vi "Sequence.CreateStepLoop.vi"(7 "Iteration":string, 8 "error in (no error)":errorcluster, 10 "Duration":dbl, 11 "Elements":T1[](array[typedef])) -> (0 "error out":errorcluster, 3 "Tasks":refnum<k24>[](array[refnum]))   [LabVIEW 2015, in "Single Station Execution.lvlib"]
uses:
  Single Station Execution.lvlib
  NationalInstruments.VeriStand.RealTimeSequenceDefinitionApi
  Main.Constants.vi
  Types/Step.Types.ctl
  Types/Channel.Properties.ctl
  Types/Compiled.StepElementProperties.ctl
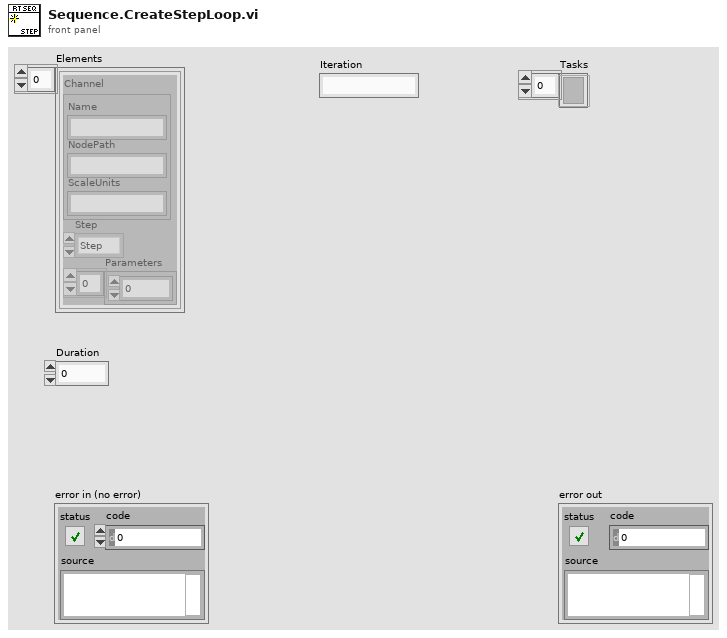
[diagram p1: front panel]
types:
  T1 = typedef "Single Station Execution.lvlib/Compiled.StepElementProperties.ctl" = cluster{"Channel":T2, "Step":T3, "Parameters":dbl[]}
  T2 = typedef "Single Station Execution.lvlib/Channel.Properties.ctl" = cluster{"Name":string, "NodePath":string, "ScaleUnits":string}
  T3 = typedef "Single Station Execution.lvlib/Step.Types.ctl" = enum8{"Step", "iStep", "Ramp", "Unchanged", "Unknown", "Sine", "LogSine", "LinearSine", "ForcedRamp", "Waveform"}
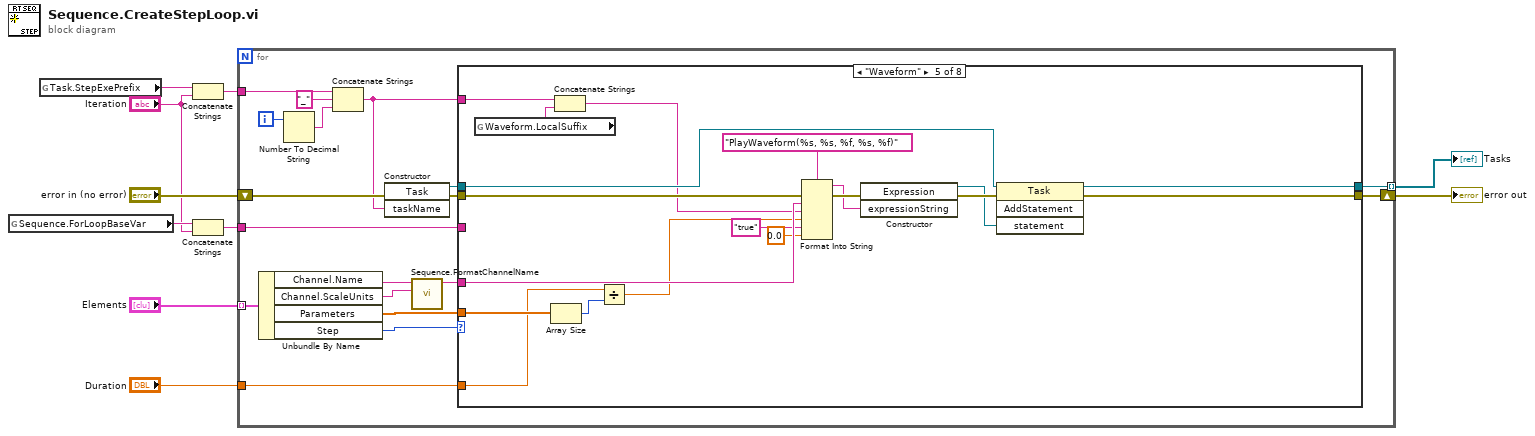
[diagram p0: block diagram]
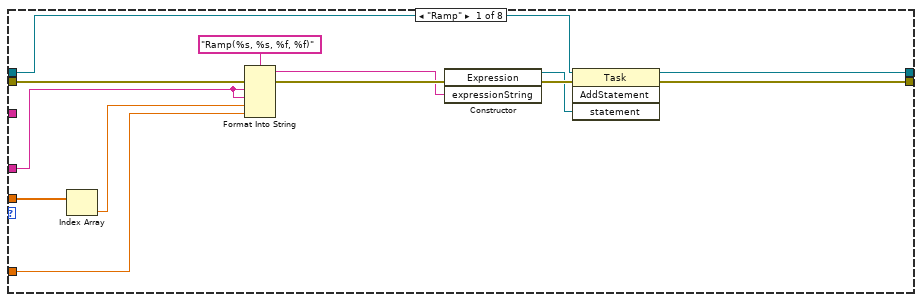
[diagram p2: hidden frame]
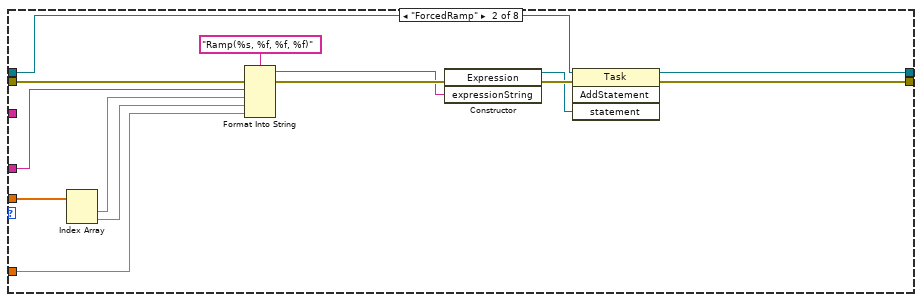
[diagram p3: hidden frame]
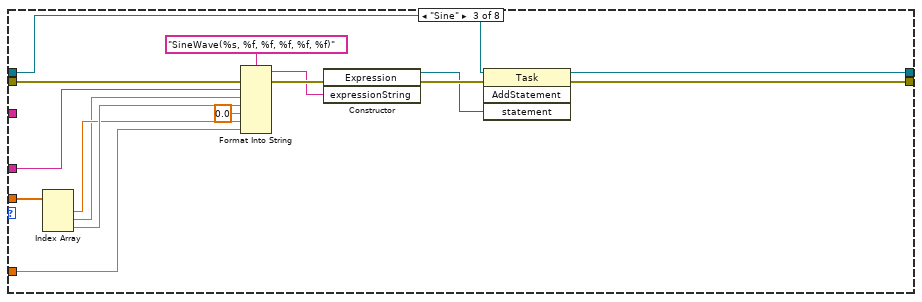
[diagram p4: hidden frame]
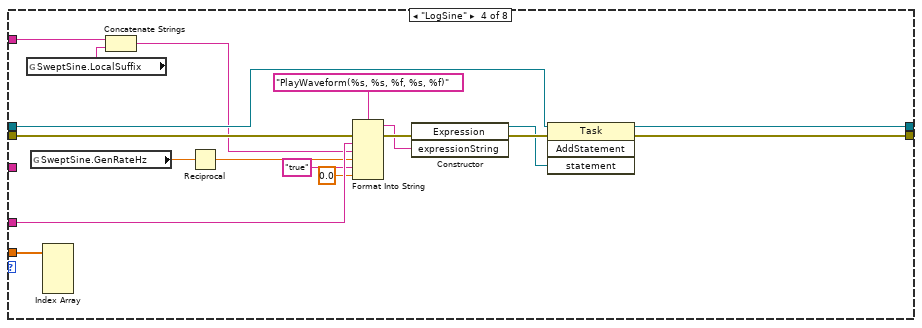
[diagram p5: hidden frame]
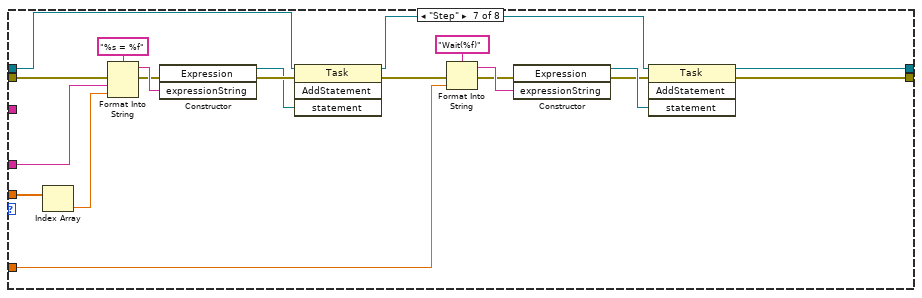
[diagram p7: hidden frame]
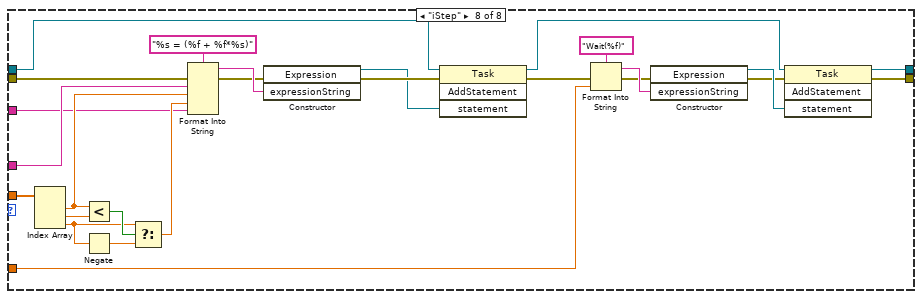
[diagram p8: hidden frame]
diagram:
  n1 = global read "Main.Constants.vi" "Sequence.ForLoopBaseVar"() -> (w3:string)
  n2 = global read "Main.Constants.vi" "Task.StepExePrefix"() -> (w5:string)
  n3 = Concatenate Strings(w5, "Iteration") -> (w4:string)
  n4 = Concatenate Strings(w3, "Iteration") -> (w1:string)
  n5 = for {
    tunnel: "Elements" -> [w24] mode=indexing
    shift-right: [w15] -> w9
    shift-left: "error in (no error)" -> [w23]
    tunnel: w4 -> [w27]
    tunnel: [w13] -> w10 mode=indexing
    tunnel: "Duration" -> [w19]
    tunnel: w1 -> [w12]
    i -> [w28]
    n6 = Unbundle By Name(w24) -> ("Channel.Name"=w22:string, "Channel.ScaleUnits"=w21:string, "Parameters"=w18:dbl[], "Step"=w17:T3)
    n7 = Number To Decimal String(number=w28) -> (decimal integer string=w25:string)  [unwired: 1 in]
    n8 = Concatenate Strings(w27, "_" ("string"), w25) -> (w11:string)
    n9 = constructor class="Task"(error in=w23, "taskName"=w11) -> (reference out=w14:refnum<k24>, error out=w16:errorcluster)  [unwired: 2 in, 2 out]
    n10 = call "Sequence.FormatChannelName.vi"("ScaleUnits"=w21, "Name"=w22) -> ("ChannelName"=w20:string)  [unwired: 9 in]
    n11 = case shown="\"Waveform\"" w17 {
      tunnel: w20 -> [w41 w55 w70 w88 w107 _ w129 w155]
      tunnel: w18 -> [w30 w43 w69 w87 w92 _ w128 w154]
      tunnel: w19 -> [w39 w52 w58 _ w90 _ w119 w146]
      tunnel: [w33 w46 w63 w81 w101 w109 w113 w140] -> w15
      tunnel: w16 -> [w38 w51 w68 w86 w106 w109 w126 w153]
      tunnel: w14 -> [w35 w48 w65 w83 w103 w110 w118 w145]
      tunnel: [w32 w45 w62 w80 w100 w110 w111 w138] -> w13
      tunnel: w12 -> [_ _ _ _ _ _ _ w131]
      tunnel: w11 -> [_ _ _ w75 w96 _ _ _]
      frame "Ramp" {
        n12 = Index Array(array=w30) -> (element=w40:dbl)  [unwired: 1 in]
        n13 = Format Into String(format string="Ramp(%s, %s, %f, %f)" ("expressionString"), error in=w38, w41, w41, w40, w39) -> (resulting string=w31:string, error out=w34:errorcluster)  [unwired: 1 in]
        n14 = constructor class="Expression"(error in=w34, "expressionString"=w31) -> (reference out=w36:refnum<k24>, error out=w37:errorcluster)  [unwired: 2 in, 2 out]
        n15 = invoke class="Task" method="AddStatement"(reference=w35, error in=w37, "statement"=w36) -> (reference out=w32:refnum<k24>, error out=w33:errorcluster)  [unwired: 1 in, 2 out]
      }
      frame "ForcedRamp" {
        n16 = Index Array(array=w43) -> (element #1=w54:dbl, element #2=w53:dbl)  [unwired: 2 in]
        n17 = Format Into String(format string="Ramp(%s, %f, %f, %f)" ("expressionString"), error in=w51, w55, w54, w53, w52) -> (resulting string=w44:string, error out=w47:errorcluster)  [unwired: 1 in]
        n18 = constructor class="Expression"(error in=w47, "expressionString"=w44) -> (reference out=w49:refnum<k24>, error out=w50:errorcluster)  [unwired: 2 in, 2 out]
        n19 = invoke class="Task" method="AddStatement"(reference=w48, error in=w50, "statement"=w49) -> (reference out=w45:refnum<k24>, error out=w46:errorcluster)  [unwired: 1 in, 2 out]
      }
      frame "Sine" {
        n20 = Index Array(array=w69) -> (element #1=w57:dbl, element #2=w56:dbl, element #3=w60:dbl)  [unwired: 3 in]
        n21 = Format Into String(format string="SineWave(%s, %f, %f, %f, %f, %f)" ("expressionString"), error in=w68, w70, w56, w60, 0.0 ("input 4"), w57, w58) -> (resulting string=w61:string, error out=w64:errorcluster)  [unwired: 1 in]
        n22 = constructor class="Expression"(error in=w64, "expressionString"=w61) -> (reference out=w66:refnum<k24>, error out=w67:errorcluster)  [unwired: 2 in, 2 out]
        n23 = invoke class="Task" method="AddStatement"(reference=w65, error in=w67, "statement"=w66) -> (reference out=w62:refnum<k24>, error out=w63:errorcluster)  [unwired: 1 in, 2 out]
      }
      frame "LogSine" {
        n24 = global read "Main.Constants.vi" "SweptSine.LocalSuffix"() -> (w73:string)
        n25 = global read "Main.Constants.vi" "SweptSine.GenRateHz"() -> (w72:dbl)
        n26 = Index Array(array=w87) -> ()  [unwired: 4 in, 4 out]
        n27 = Concatenate Strings(w75, w73) -> (w74:string)
        n28 = Reciprocal(x=w72) -> (1/x=w76:dbl)
        n29 = Format Into String(format string="PlayWaveform(%s, %s, %f, %s, %f)" ("expressionString"), error in=w86, w88, w74, w76, "true" ("input 4"), 0.0 ("input 4")) -> (resulting string=w79:string, error out=w82:errorcluster)  [unwired: 1 in]
        n30 = constructor class="Expression"(error in=w82, "expressionString"=w79) -> (reference out=w84:refnum<k24>, error out=w85:errorcluster)  [unwired: 2 in, 2 out]
        n31 = invoke class="Task" method="AddStatement"(reference=w83, error in=w85, "statement"=w84) -> (reference out=w80:refnum<k24>, error out=w81:errorcluster)  [unwired: 1 in, 2 out]
      }
      frame "Waveform" {
        n32 = global read "Main.Constants.vi" "Waveform.LocalSuffix"() -> (w94:string)
        n33 = Array Size(array=w92) -> (size(s)=w93:i32)
        n34 = Concatenate Strings(w96, w94) -> (w95:string)
        n35 = Divide(x=w90, y=w93) -> (x/y=w91:dbl)
        n36 = Format Into String(format string="PlayWaveform(%s, %s, %f, %s, %f)" ("expressionString"), error in=w106, w107, w95, w91, "true" ("input 4"), 0.0 ("input 4")) -> (resulting string=w99:string, error out=w102:errorcluster)  [unwired: 1 in]
        n37 = constructor class="Expression"(error in=w102, "expressionString"=w99) -> (reference out=w104:refnum<k24>, error out=w105:errorcluster)  [unwired: 2 in, 2 out]
        n38 = invoke class="Task" method="AddStatement"(reference=w103, error in=w105, "statement"=w104) -> (reference out=w100:refnum<k24>, error out=w101:errorcluster)  [unwired: 1 in, 2 out]
      }
      frame "Unchanged", Default {
      }
      frame "Step" {
        n39 = Index Array(array=w128) -> (element=w127:dbl)  [unwired: 1 in]
        n40 = Format Into String(format string="%s = %f" ("expressionString"), error in=w126, w129, w127) -> (resulting string=w123:string, error out=w114:errorcluster)  [unwired: 1 in]
        n41 = constructor class="Expression"(error in=w114, "expressionString"=w123) -> (reference out=w124:refnum<k24>, error out=w125:errorcluster)  [unwired: 2 in, 2 out]
        n42 = invoke class="Task" method="AddStatement"(reference=w118, error in=w125, "statement"=w124) -> (reference out=w112:refnum<k24>, error out=w115:errorcluster)  [unwired: 1 in, 2 out]
        n43 = Format Into String(format string="Wait(%f)", error in=w115, w119) -> (resulting string=w117:string, error out=w116:errorcluster)  [unwired: 1 in]
        n44 = constructor class="Expression"(error in=w116, "expressionString"=w117) -> (reference out=w122:refnum<k24>, error out=w121:errorcluster)  [unwired: 2 in, 2 out]
        n45 = invoke class="Task" method="AddStatement"(reference=w112, error in=w121, "statement"=w122) -> (reference out=w111:refnum<k24>, error out=w113:errorcluster)  [unwired: 1 in, 2 out]
      }
      frame "iStep" {
        n46 = Index Array(array=w154) -> (element #1=w137:dbl, element #2=w136:dbl, element #3=w133:dbl)  [unwired: 3 in]
        n47 = Less?(x=w137, y=w136) -> (x < y?=w135:bool)
        n48 = Negate(x=w133) -> (-x=w134:dbl)
        n49 = Select(t=w133, s=w135, f=w134) -> (s? t:f=w132:dbl)
        n50 = Format Into String(format string="%s = (%f + %f*%s)" ("expressionString"), error in=w153, w155, w137, w132, w131) -> (resulting string=w150:string, error out=w141:errorcluster)  [unwired: 1 in]
        n51 = constructor class="Expression"(error in=w141, "expressionString"=w150) -> (reference out=w151:refnum<k24>, error out=w152:errorcluster)  [unwired: 2 in, 2 out]
        n52 = invoke class="Task" method="AddStatement"(reference=w145, error in=w152, "statement"=w151) -> (reference out=w139:refnum<k24>, error out=w142:errorcluster)  [unwired: 1 in, 2 out]
        n53 = Format Into String(format string="Wait(%f)", error in=w142, w146) -> (resulting string=w144:string, error out=w143:errorcluster)  [unwired: 1 in]
        n54 = constructor class="Expression"(error in=w143, "expressionString"=w144) -> (reference out=w149:refnum<k24>, error out=w148:errorcluster)  [unwired: 2 in, 2 out]
        n55 = invoke class="Task" method="AddStatement"(reference=w139, error in=w148, "statement"=w149) -> (reference out=w138:refnum<k24>, error out=w140:errorcluster)  [unwired: 1 in, 2 out]
      }
    }
  }
  "Tasks" <- w10
  "error out" <- w9
